vi "Define Units.vi"(8 "error in":errorcluster, 11 "analog channel in":refnum<class "Analog Channel.lvclass">) -> (0 "error out":errorcluster, 3 "analog channel out":refnum<class "Analog Channel.lvclass">)   [LabVIEW 2020, in "Scan Engine Scripting.lvlib" / "Analog Channel.lvclass"]
uses:
  Analog Channel.lvclass
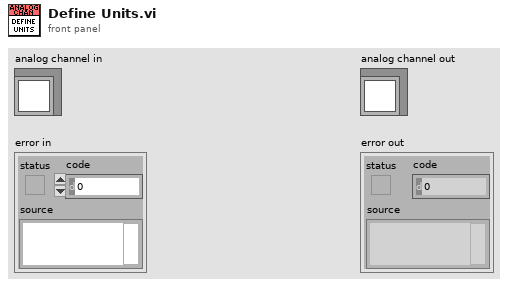
[diagram p1: front panel]
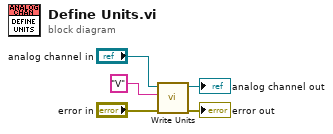
[diagram p0: block diagram]
diagram:
  n1 = call-dynamic "Write Units.vi"("error in"="error in", "units"="V", "channel in"="analog channel in") -> ("error out"=→"error out":errorcluster, "channel out"=→"analog channel out":refnum<class "Analog Channel.lvclass">)  [unwired: 7 in]
